vi "StringToConstant Array.vi"(11 "String Constant Array In":string[](array[string])) -> (3 "I32 Constant Array Out":i32[](array[numeric]))   [LabVIEW 2021]
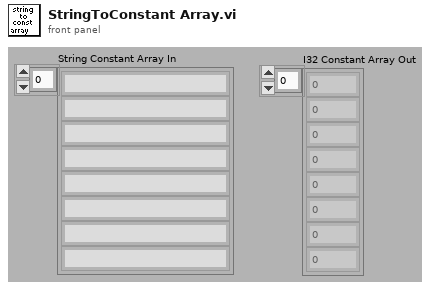
[diagram p1: front panel]
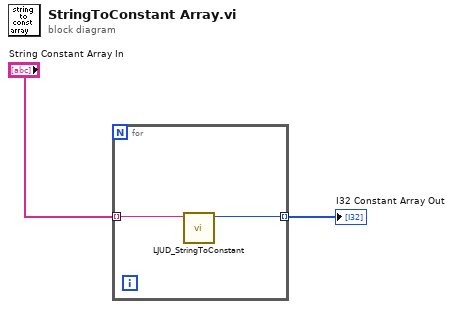
[diagram p0: block diagram]
diagram:
  n1 = for {
    tunnel: "String Constant Array In" -> [w4] mode=indexing
    tunnel: [w3] -> w1 mode=indexing
    n2 = call "LJUD_StringToConstant.vi"("String"=w4) -> ("Constant Number"=w3:i32)  [unwired: 9 in, 1 out]
  }
  "I32 Constant Array Out" <- w1
